vi "Read Will Info.vi"(8 "error in (no error)":errorcluster, 11 "mqtt in":refnum<class "MQTT Client.lvclass">) -> (0 "error out":errorcluster, 2 "Will Info":T1={"Will message"="Last Will", "Will Topic"="Will Topic"}, 3 "mqtt out":refnum<class "MQTT Client.lvclass">)   [LabVIEW 2020, in "MQTT Client.lvclass"]
uses:
  MQTT Client.lvclass
  mqttTypedef/mqttWillInfo.ctl
  MQTT Client.lvclass/MQTT Client.ctl
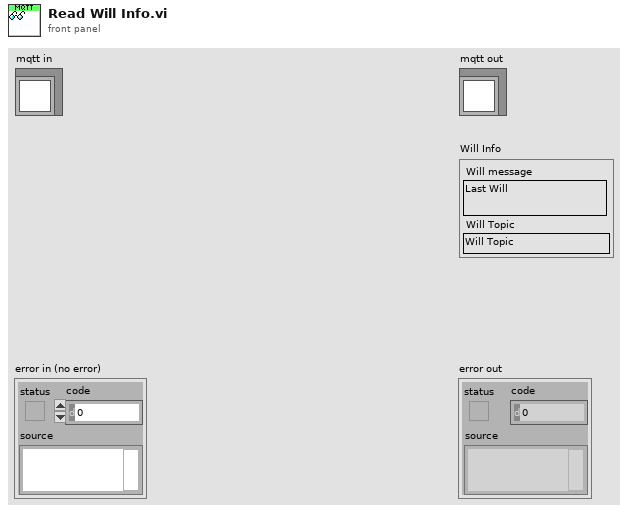
[diagram p1: front panel]
types:
  T1 = typedef "MQTT Client.lvclass/mqttWillInfo.ctl" = cluster{"Will message":string, "Will Topic":string}
  T2 = typedef "mqtt.lvclass/mqttWillInfo.ctl" = cluster{"Will message":string, "Will Topic":string}
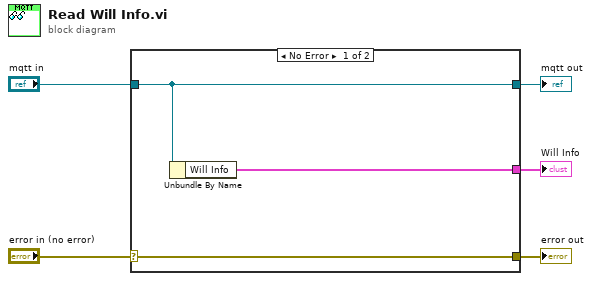
[diagram p0: block diagram]
diagram:
  n1 = case shown="No Error" "error in (no error)" {
    selector: "error in (no error)" -> [w8 w9]
    tunnel: [w8 w9] -> w4
    tunnel: [w7 w10] -> w2
    tunnel: "mqtt in" -> [w7 w10]
    tunnel: [w6 _] -> w1
    frame No Error {
      n2 = Unbundle By Name(w7) -> ("Will Info"=w6:T2)
    }
    frame Error {
    }
  }
  "error out" <- w4
  "mqtt out" <- w2
  "Will Info" <- w1
